vi "Set Diverter.vi"(8 "error in (no error)":errorcluster, 9 "Diverter Port":T1, 10 "Diverter Location":T2, 11 "Abstract Spectrometer in":refnum<class "Abstract Spectrometer.lvclass">) -> (0 "error out":errorcluster, 1 "Diverter Port out":T1, 3 "Abstract Spectrometer out":refnum<class "Abstract Spectrometer.lvclass">)   [LabVIEW 2019, in "Abstract Spectrometer.lvclass"]
uses:
  Abstract Spectrometer.lvclass
  SpectraPro-LabVIEW-Driver/Libraries/Types/Diverter Location.ctl
  SpectraPro-LabVIEW-Driver/Libraries/Types/Diverter Port.ctl
  SpectraPro-LabVIEW-Driver/SpectraPro.lvlib
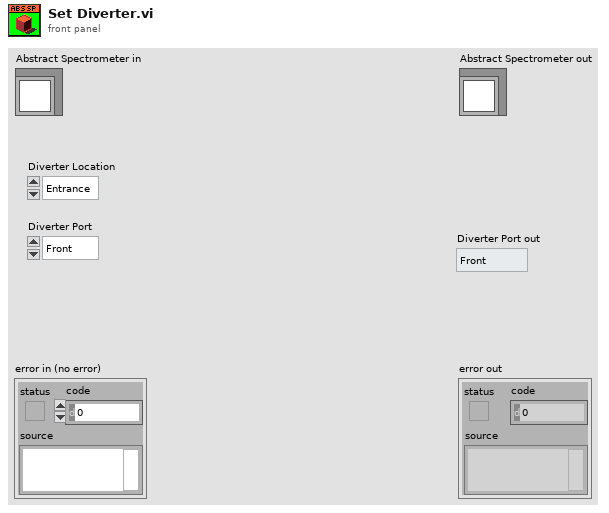
[diagram p1: front panel]
types:
  T1 = typedef "SpectraPro.lvlib/Diverter Port.ctl" = enum16{"Front", "Side"}
  T2 = typedef "Diverter Location.ctl" = enum16{"Entrance", "Exit"}
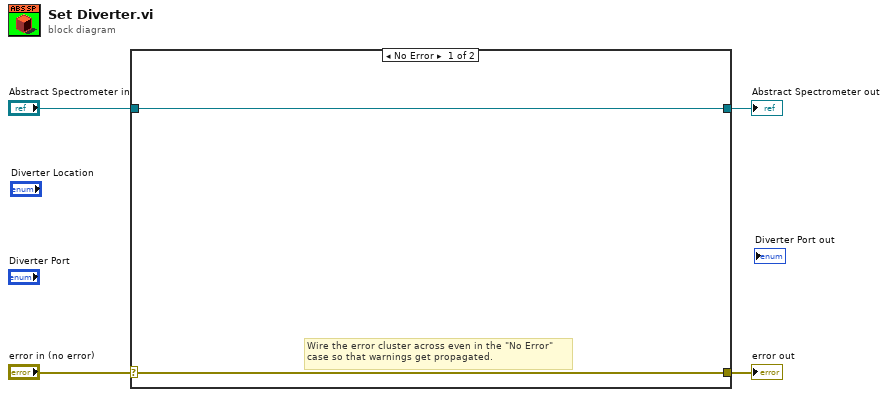
[diagram p0: block diagram]
diagram:
  n1 = case shown="No Error" "error in (no error)" {
    selector: "error in (no error)" -> [w5 w8]
    tunnel: [w5 w8] -> w3
    tunnel: [w6 w7] -> w1
    tunnel: "Abstract Spectrometer in" -> [w6 w7]
    frame No Error {
      # "Wire the error cluster across even in the \"No Error\"\ncase so that warnings get propagated."
    }
    frame Error {
    }
  }
  "error out" <- w3
  "Abstract Spectrometer out" <- w1
